vi "TDT-Sampling Rate to LoadCOFsf Input.vi"(7 "Sampling rate (Hz)":dbl) -> (8 "LoadCOFsf Input":dbl)   [LabVIEW 2020]
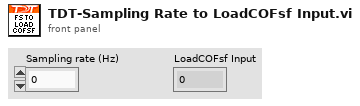
[diagram p1: front panel]
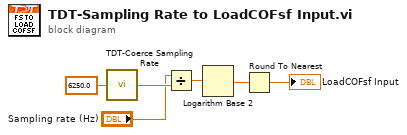
[diagram p0: block diagram]
diagram:
  n1 = call "TDT-Coerce Sampling Rate.vi"("Fs (Hz)"=6250.0) -> ("Coerced"=w3:dbl)
  n2 = Divide(x="Sampling rate (Hz)", y=w3) -> (x/y=w4:dbl)
  n3 = Logarithm Base 2(1:w4) -> (0:w5:dbl)
  n4 = Round To Nearest(number=w5) -> (nearest integer value=→"LoadCOFsf Input":dbl)
